vi "Get Results - ArrayOfClusters.vi"(8 "error in (no error)":errorcluster, 10 "Input Operations":T2(array[cluster]), 11 "Array":T1(array[cluster])) -> (0 "error out":errorcluster, 2 "Output Operations":T2(array[cluster]), 3 "output array":T1(array[cluster]))   [LabVIEW 2011]
uses:
  ClassDefinitions/SimpleClassWithMethods/SimpleArithmetic.lvclass
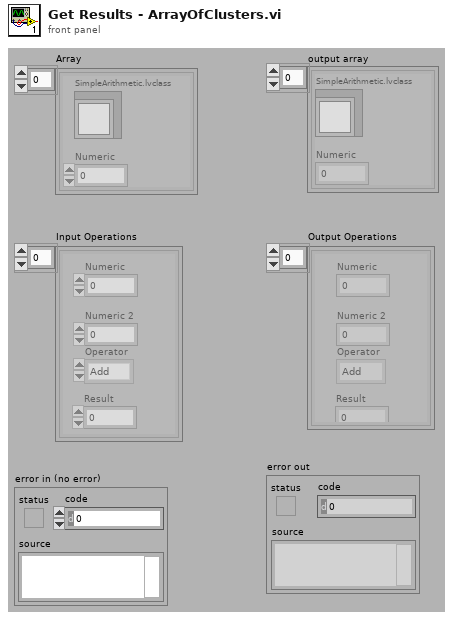
[diagram p1: front panel]
types:
  T1 = cluster{"SimpleArithmetic.lvclass":refnum<class "SimpleArithmetic.lvclass">, "Numeric":dbl}[]
  T2 = cluster{"Numeric":dbl, "Numeric 2":dbl, "Operator":enum16{"Add", "Divide", "Multiple", "Subtract"}, "Result":dbl}[]
  T3 = cluster{"SimpleArithmetic.lvclass":refnum<class "SimpleArithmetic.lvclass">, "Numeric":dbl}
  T4 = cluster{"Numeric":dbl, "Numeric 2":dbl, "Operator":enum16{"Add", "Divide", "Multiple", "Subtract"}, "Result":dbl}
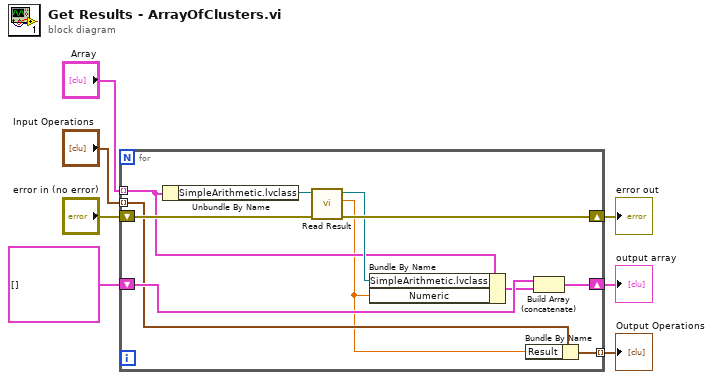
[diagram p0: block diagram]
diagram:
  n1 = for {
    tunnel: "Array" -> [w9] mode=indexing
    tunnel: "Input Operations" -> [w14] mode=indexing
    shift-right: [w15] -> w1
    shift-left: T1 [] ("Array") -> [w17]
    shift-right: [w16] -> w5
    shift-left: "error in (no error)" -> [w18]
    tunnel: [w13] -> w4 mode=indexing
    n2 = Unbundle By Name(w9) -> ("SimpleArithmetic.lvclass"=w12:refnum<class "SimpleArithmetic.lvclass">)
    n3 = call "Read Result.vi"("error in (no error)"=w18, "SimpleArithmetic in"=w12) -> ("error out"=w16:errorcluster, "Result"=w8:dbl, "SimpleArithmetic out"=w10:refnum<class "SimpleArithmetic.lvclass">)  [unwired: 7 in]
    n4 = Bundle By Name(cluster=w9, "SimpleArithmetic.lvclass"=w10, "Numeric"=w8) -> (w11:T3)
    n5 = Bundle By Name(cluster=w14, "Result"=w8) -> (w13:T4)
    n6 = Build Array (concatenate)(w17, w11) -> (w15:T1)
  }
  "error out" <- w5
  "Output Operations" <- w4
  "output array" <- w1
